vi "PH_gentec_Powermeter.constructor.vi"(0 "name":string, 2 "data in":string, 5 "error in":errorcluster) -> (14 "i ref out":refnum<vi>, 16 "data out":string, 19 "error out":errorcluster)   [LabVIEW 2014, in "PH_gentec_Powermeter.lvlib"]
doc: "This class is forseen to control a gentec powermeter.\n\nThis class is part of the PHELIX device layer.\n\nauthor: Andreas Meidrott, GSI\n\nLicense Agreement for this software:\n\nCopyright (C)\nGesellschaft für Schwerionenforschung, GSI\nPlanckstr. 1\n64291 Darmstadt\nGermany\n\nContact: D.Beck@gsi.de \n\nThis program is free software; you can redistribute it and/or modify it under the terms of the \nGNU General Public License as published by the Free Software Foundation; either version 2 of \nthe license, or (at your option) any later version.\n\nThis program is distributed in the hope that it will be useful, but WITHOUT ANY WARRANTY; \nwithout even the implied warranty of MERCHANTABILITY or FITNESS FOR A PARTICULAR PURPOSE. See the GNU General License for more details (http://www.gnu.org).\n\nGesellschaft für Schwerionenforschung, GSI\nPlanckstr. 1, 64291 Darmstadt, Germany\nFor all questions and ideas contact: M.Richter@gsi.de, H.Brand@gsi.de or D.Beck@gsi.de.\nLast update: 16-JUN-2004"
uses:
  PH_gentec_Powermeter.lvlib
  PH_Basics/PH_Powermeter_BaseClass/PH_Powermeter_BaseClass.State.ctl
  PH_Basics/PH_Class/PH_Class.lvlib
  PH_Basics/PH_Powermeter_BaseClass/PH_Powermeter_BaseClass.lvlib
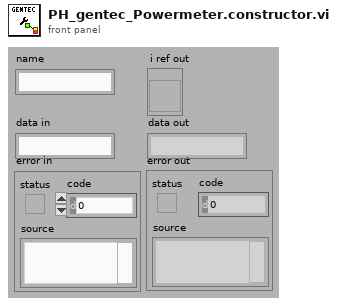
[diagram p1: front panel]
types:
  T1 = typedef "PH_Powermeter_BaseClass.lvlib/PH_Powermeter_BaseClass.State.ctl" = enum32{"off", "operating", "opened", "checked", "connected", "Sets to change", "running"}
  T2 = enum16{"SetAttribute", "GetAttribute", "CreateAttribute", "DestroyAttribute", "DestroyAllAtributes"}
  T3 = typedef "PH_gentec_Powermeter.lvlib/PH_gentec_Powermeter.i attribute.ctl" = cluster{"GUI References":cluster{"delete":refnum<vi>, "start stop Statistics":refnum<vi>, "Statistic Data":refnum<vi>, "Configuration Values":refnum<vi>, "Set Zero":refnum<vi>, "Data Sampling Settings":refnum<vi>, "Wanted Sets":refnum<vi>, "Current Sets":refnum<vi>}, "Start Stop Statistics":bool, "Wanted Sets":T4, "Current Sets":T4}
  T4 = typedef "PH_gentec_Powermeter.lvlib/PH_gentec_Powermeter.Sets.ctl" = cluster{"Data Sampling Settings":T5, "Set Zero":bool}
  T5 = typedef "gentec-SOLO-PE - Driver.lvlib/gentec-SOLO-PE.Data Sampling Settings.ctl" = cluster{"Sample Rate":u32, "Sample Rate Unit":u32, "Sample Period":u32, "Sample Period Unit":u32, "Total Duration":u32, "Total Duration Unit":u32, "Time Stamp":u32}
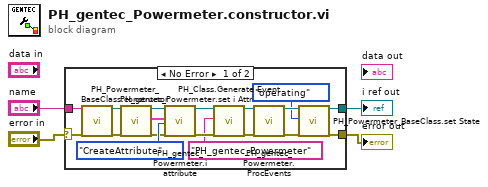
[diagram p0: block diagram]
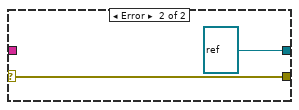
[diagram p2: hidden frame]
diagram:
  n1 = case shown="No Error" "error in" {
    selector: "error in" -> [w8 w24]
    tunnel: "name" -> [w9 _]
    tunnel: [w22 refnum<vi> refnum ("i ref out")] -> w3
    tunnel: [w21 w24] -> w2
    frame No Error {
      n2 = call "PH_Powermeter_BaseClass.constructor.vi"("name"=w9, "error in"=w8) -> ("i ref out"=w10:refnum<vi>, "error out"=w11:errorcluster)  [unwired: 15 in, 1 out]
      n3 = call "PH_gentec_Powermeter.set i Attr.vi"("i ref in"=w10, "error in"=w11) -> ("i ref out"=w14:refnum<vi>, "i Attributes"=w13:T3, "error out"=w12:errorcluster)  [unwired: 15 in]
      n4 = call "PH_gentec_Powermeter.i attribute.vi"("VI Refnum"=w14, "CLASS.i attribute"=w13, "Action"=T2."CreateAttribute", "error in (no error)"=w12) -> ("VI Refnum out"=w19:refnum<vi>, "error out"=w17:errorcluster)  [unwired: 13 in, 1 out]
      n5 = call "PH_Class.Generate Event.vi"("i ref in"=w19, "Class"="PH_gentec_Powermeter", "error in (no error)"=w17) -> ("i ref out"=w18:refnum<vi>, "error out"=w15:errorcluster)  [unwired: 15 in]
      n6 = call "PH_gentec_Powermeter.ProcEvents.vi"("i ref in"=w18, "error in"=w15) -> ("i ref out"=w7:refnum<vi>, "error out"=w6:errorcluster)  [unwired: 16 in]
      n7 = call "PH_Powermeter_BaseClass.set State.vi"("VI in"=w7, "State"=PH_Powermeter_BaseClass.State."operating", "error in (no error)"=w6) -> ("VI out"=w22:refnum<vi>, "error out"=w21:errorcluster)  [unwired: 15 in]
    }
    frame Error {
    }
  }
  "i ref out" <- w3
  "error out" <- w2
